vi "XYStage.MoveStarted.vi"(8 "error in (no error)":errorcluster, 11 "XYStage":refnum<class "XYStage.lvclass">) -> (0 "error out":errorcluster, 3 "XYStage out":refnum<class "XYStage.lvclass">)   [LabVIEW 2013, in "XYStage.lvclass"]
doc: "---------------------------------------------------------------\nJKI State Machine Objects™\nhttp://jki.net/state-machine-objects/\nCopyright (C) 2005-2015, JKI <info@jki.net>\nALL RIGHTS RESERVEDJKI State Machine Objects (SMO) 1.0.0.4\nJKI - JKI\nCopyright (c) 2015, JKI"
uses:
  XYStage.lvclass
panel:
  # "For instructions on how to use the JKI State Machine Objects, examples and video tutorials, visit:\nhttp://jki.net/state-machine-objects/\n\nJKI State Machine Objects™\nhttp://jki.net/state-machine-objects/\nCopyright (C) 2005-2015, JKI <info@jki.net>\nALL RIGHTS RESERVED"
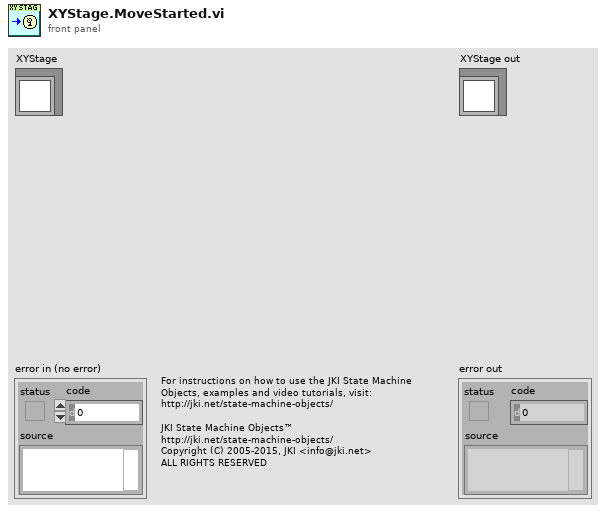
[diagram p1: front panel]
types:
  T1 = typedef "XYStage.lvclass/PrivateData--Ref.ctl" = refnum<data-value>
  T2 = typedef "XYStage.lvclass/PrivateData--Cluster.ctl" = cluster{"Dependencies":T3, "Public Events":T4, "Protected Events":T5, "Private Events":T6, "Configuration":T7, "Target":T8, "Move Parameters":T11}
  T3 = typedef "XYStage.lvclass/Dependencies--Cluster.ctl" = cluster{"Positions":refnum<class "SMO.Dictionary.Variant.lvclass">}
  T4 = typedef "XYStage.lvclass/PublicEvents--Cluster.ctl" = cluster{"MoveComplete":refnum<user-event>, "NewPosition":refnum<user-event>, "UpdatedNamedPosition":refnum<user-event>, "MoveStarted":refnum<user-event>}
  T5 = typedef "XYStage.lvclass/ProtectedEvents--Cluster.ctl" = cluster{"API_Template":refnum<user-event>}
  T6 = typedef "XYStage.lvclass/PrivateEvents--Cluster.ctl" = cluster{"MoveAbsolute":refnum<user-event>, "MoveRelative":refnum<user-event>, "MoveToNamedPosition":refnum<user-event>, "StorePosition":refnum<user-event>, "Home":refnum<user-event>}
  T7 = typedef "XYStage.lvclass/Configuration--Cluster.ctl" = cluster{"Real-World Units":string, "Counts per Unit":dbl}
  T8 = typedef "XYStage.lvclass/TargetPositions--Cluster.ctl" = cluster{"Coords":T9, "Counts":T10}
  T9 = typedef "XYStage.lvclass/(real)Coords--Cluster.ctl" = cluster{"X":dbl, "Y":dbl}
  T10 = typedef "XYStage.lvclass/(counts)Coords--Cluster.ctl" = cluster{"X":i32, "Y":i32}
  T11 = typedef "XYStage.lvclass/MoveParameters--Cluster.ctl" = cluster{"Velocity (units/s)":dbl, "Acceleration (units/s^2)":dbl}
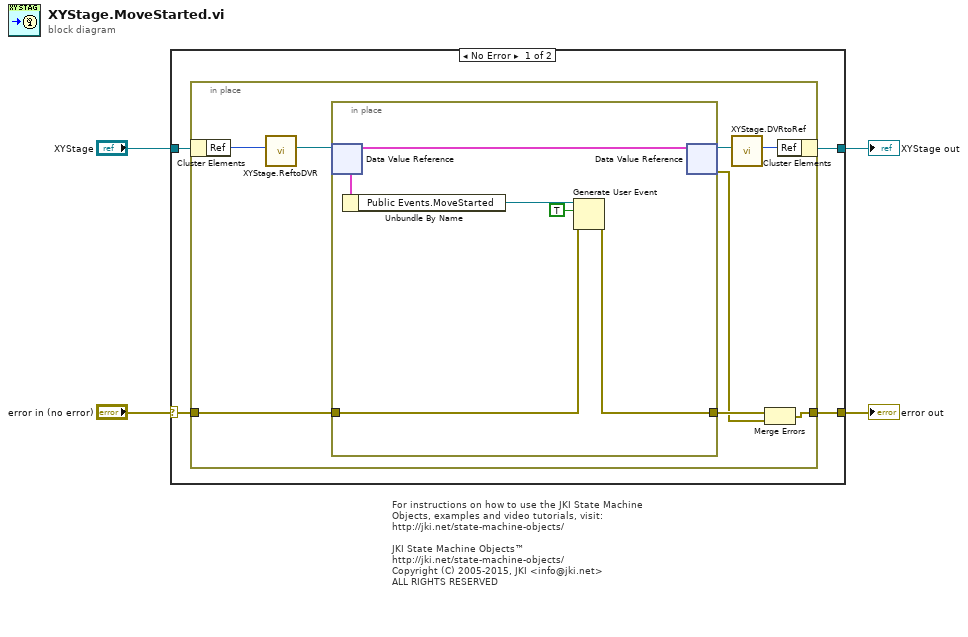
[diagram p0: block diagram]
diagram:
  # "For instructions on how to use the JKI State Machine Objects, examples and video tutorials, visit:\nhttp://jki.net/state-machine-objects/\n\nJKI State Machine Objects™\nhttp://jki.net/state-machine-objects/\nCopyright (C) 2005-2015, JKI <info@jki.net>\nALL RIGHTS RESERVED"
  n1 = case shown="No Error" "error in (no error)" {
    selector: "error in (no error)" -> [w6 w23]
    tunnel: [w5 w23] -> w3
    tunnel: [w7 w22] -> w4
    tunnel: "XYStage" -> [w8 w22]
    frame No Error {
      n2 = in-place {
        in-place-border: w6 -> [w16]
        in-place-border: [w13] -> w5
        n3 = in-place-cluster #1(w8) -> ("Ref"=w12:u32)
        n4 = call "XYStage.ReftoDVR.vi"("Ref"=w12) -> ("Ref"=w10:T1)  [unwired: 10 in]
        n5 = in-place {
          in-place-border: w16 -> [w20]
          in-place-border: [w19] -> w15
          n6 = in-place-dvr #2(w10) -> (w17:T2)  [unwired: 1 out]
          n7 = Unbundle By Name(w17) -> ("Public Events.MoveStarted"=w21:refnum<user-event>)
          n8 = Generate User Event(user event=w21, event data cluster=TRUE ("event data"), error in=w20) -> (error out=w19:errorcluster)  [unwired: 1 in, 1 out]
          n9 = in-place-dvr #2(w17) -> (w11:T1, w14:errorcluster)
        }
        n10 = call "XYStage.DVRtoRef.vi"("Ref"=w11) -> ("Ref"=w9:u32)  [unwired: 10 in]
        n11 = Merge Errors(w15, w14) -> (w13:errorcluster)
        n12 = in-place-cluster #1("Ref"=w9) -> (w7:refnum<class "XYStage.lvclass">)
      }
    }
    frame Error {
    }
  }
  "error out" <- w3
  "XYStage out" <- w4
